vi "RPC Method hello_hi.vi"(8 "error in (no error)":errorcluster, 10 "Request Data":T2, 11 "gRPC Client in":refnum<class "Simple_client.lvclass">) -> (0 "error out":errorcluster, 2 "Response Data":T1, 3 "gRPC Client out":refnum<class "Simple_client.lvclass">)   [LabVIEW 2019, in "Simple_client.lvlib" / "Simple_client.lvclass"]
uses:
  Simple_client.lvclass
  RPC Messages/simpleMsgReq/simpleMsgReq_Data.ctl
  RPC Messages/simpleMgsReply/simpleMgsReply_Data.ctl
  Simple_client.lvclass/Simple_client.ctl
  fa22ca14-33b2-4bc3-8699-3f27c9b27c9c.vi
  <vilib>/gRPC/LabVIEW gRPC Library/Server API/Server/Get Server DLL Path.vi
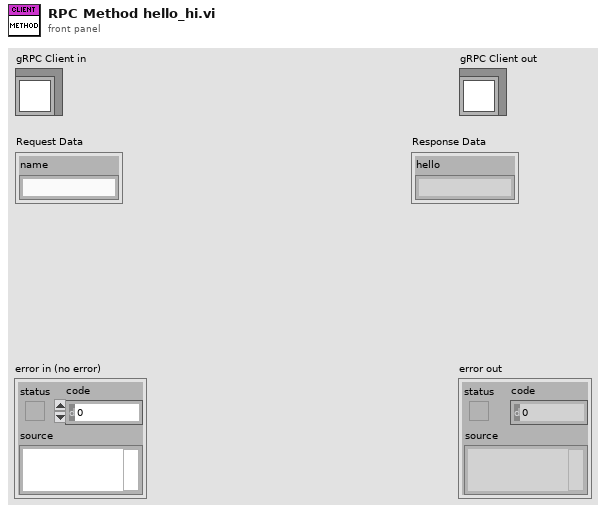
[diagram p1: front panel]
types:
  T1 = typedef "Simple_client.lvlib/Simple_client.lvclass/simpleMgsReply_Data.ctl" = cluster{"hello":string}
  T2 = typedef "Simple_client.lvlib/Simple_client.lvclass/simpleMsgReq_Data.ctl" = cluster{"name":string}
  T3 = typedef "gprc-lvsupport-release.lvlib/grpcId.ctl" = u64
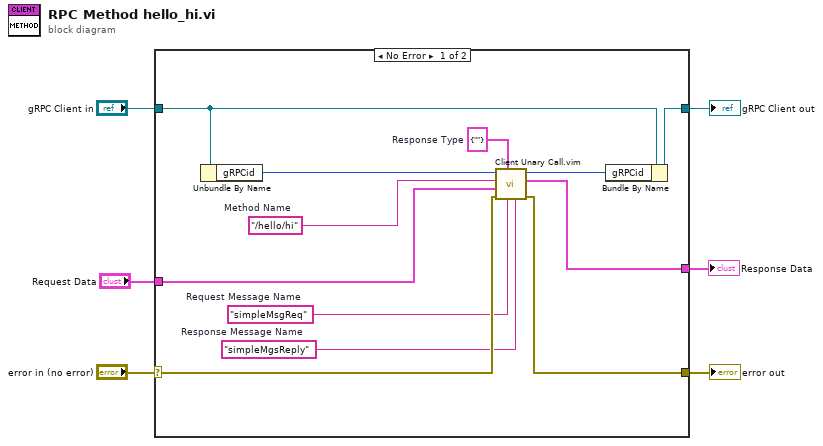
[diagram p0: block diagram]
diagram:
  n1 = case shown="No Error" "error in (no error)" {
    selector: "error in (no error)" -> [w14 w20]
    tunnel: [w13 w20] -> w5
    tunnel: [w15 w19] -> w3
    tunnel: "gRPC Client in" -> [w17 w19]
    tunnel: "Request Data" -> [w11 _]
    tunnel: [w10 _] -> w1
    frame No Error {
      w7 = "simpleMgsReply"  # Response Message Name
      w8 = "simpleMsgReq"  # Request Message Name
      w9 = T1 {"hello"=""}  # Response Type
      w12 = "/hello/hi"  # Method Name
      n2 = Unbundle By Name(w17) -> ("gRPCid"=w18:T3)
      n3 = call "Client Unary Call.vim"("Response Message Name"=w7, "Request Message Name"=w8, "Response Type"=w9, "error in (no error)"=w14, "Request Data"=w11, "Method Name"=w12, "Client Ref"=w18) -> ("error out"=w13:errorcluster, "Response Data"=w10:T1, "Client Ref Out"=w16:u64)  [unwired: 2 in]
      n4 = Bundle By Name(cluster=w17, "gRPCid"=w16) -> (w15:refnum<class "Simple_client.lvclass">)
    }
    frame Error {
    }
  }
  "error out" <- w5
  "gRPC Client out" <- w3
  "Response Data" <- w1
